vi "set value.vi"(8 "error in (no error)":errorcluster, 9 "Set value":dbl, 10 "Control Name":string="Pre-Acc", 11 "VI Refnum":refnum<vi>) -> (0 "error out":errorcluster, 3 "Output string":string)   [LabVIEW 2016, in "sub-VIs.lvlib"]
doc: "Used to set value for control value of a given VI"
uses:
  sub-VIs/sub-VIs.lvlib
panel:
  out "reference out":refnum<vi>
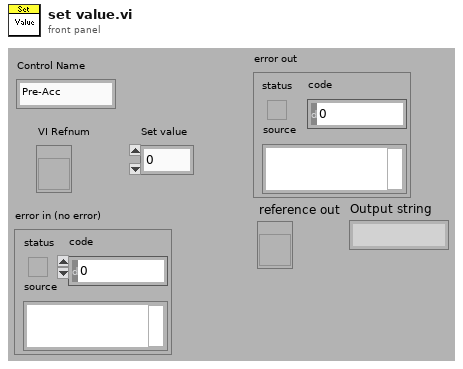
[diagram p1: front panel]
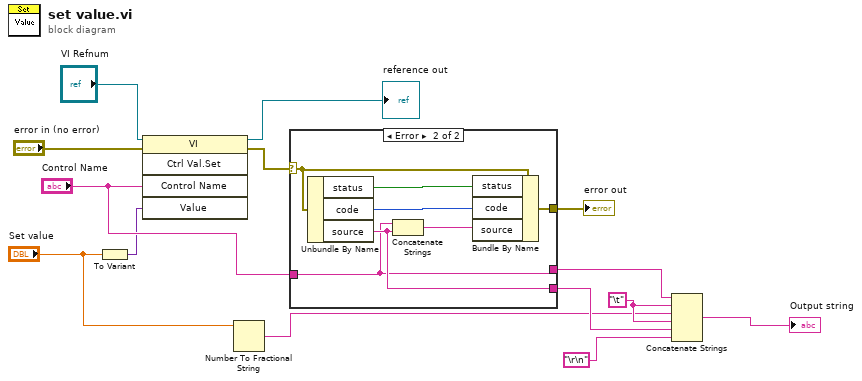
[diagram p0: block diagram]
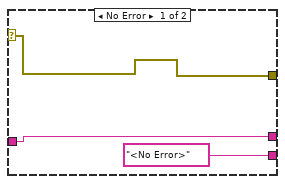
[diagram p2: hidden frame]
diagram:
  w8 = "\t"
  n1 = To Variant(anything="Set value") -> (Variant=w5:variant)
  n2 = invoke class="VI" method="Ctrl Val.Set"(reference="VI Refnum", error in="error in (no error)", "Control Name"="Control Name", "Value"=w5) -> (reference out=→"reference out":refnum<vi>, error out=w10:errorcluster)  [unwired: 1 in, 3 out]
  n3 = Number To Fractional String(number="Set value") -> (F-format string=w1:string)  [unwired: 3 in]
  n4 = case shown="Error" w10 {
    selector: w10 -> [w17 w24]
    tunnel: [w17 w21] -> w9
    tunnel: "Control Name" -> [w16 w18]
    tunnel: ["<No Error>" ("source") w19] -> w4
    tunnel: [w16 w18] -> w7
    frame No Error {
    }
    frame Error {
      n5 = Unbundle By Name(w24) -> ("status"=w23:bool, "code"=w22:i32, "source"=w19:string)
      n6 = Concatenate Strings(w18, w19) -> (w20:string)
      n7 = Bundle By Name(cluster=w24, "status"=w23, "code"=w22, "source"=w20) -> (w21:errorcluster)
    }
  }
  "error out" <- w9
  n8 = Concatenate Strings(w7, w8, w1, w8, w4, "\r\n") -> (→"Output string":string)
